vi "Write Condition.vi"(10 "Allow":i32[](array[numeric]), 11 "Interlock I32 in":refnum<class "IL I32 Pass.lvclass">) -> (3 "Interlock I32 out":refnum<class "IL I32 Pass.lvclass">)   [LabVIEW 2015, in "Interlocks.lvlib" / "IL I32 Pass.lvclass"]
uses:
  IL I32 Pass.lvclass
  IL I32 Pass.lvclass/IL I32 Pass.ctl
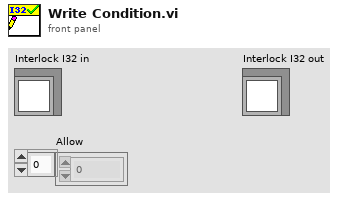
[diagram p1: front panel]
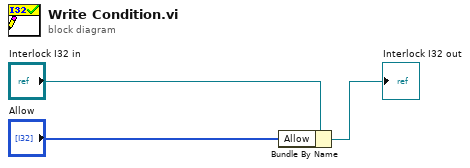
[diagram p0: block diagram]
diagram:
  n1 = Bundle By Name(cluster="Interlock I32 in", "Allow"="Allow") -> (→"Interlock I32 out":refnum<class "IL I32 Pass.lvclass">)
